vi "Remove Keys.vi"(8 "error in (no error)":errorcluster) -> (0 "error out":errorcluster, 3 "text":string)   [LabVIEW 2017, in "csm-ini-variable-addon.lvclass"]
uses:
  csm-ini-variable-addon.lvclass
  INI-Static-Variable-Support/LabVIEW-Config/LabVIEW-Config.lvclass
panel:
  out "Section Names After":string[](array[string])
  out "Key Names Before":string[](array[string])
  out "Key Names After":string[](array[string])
  out "Section Names Before":string[](array[string])
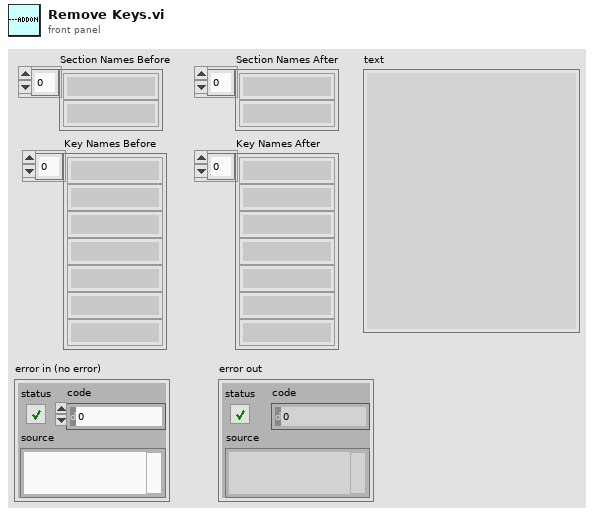
[diagram p1: front panel]
types:
  T1 = typedef "LabVIEW-Config.lvlib/LabVIEW-Config.lvclass/Config.ctl" = cluster{"Path":path, "Lines":string[], "Tokens":T2[], "Modified?":bool, "Cache":cluster{"Valid?":bool, "Key Information":T3[]}}
  T2 = typedef "LabVIEW-Config.lvlib/LabVIEW-Config.lvclass/LineToken.ctl" = enum8{"comment", "section", "key", "more"}
  T3 = typedef "LabVIEW-Config.lvlib/LabVIEW-Config.lvclass/KeyInfo.ctl" = cluster{"Key Indexes":cluster{"Indexes":i32[]}[], "Session Found?":bool, "Key found?":bool, "Session Index":i32}
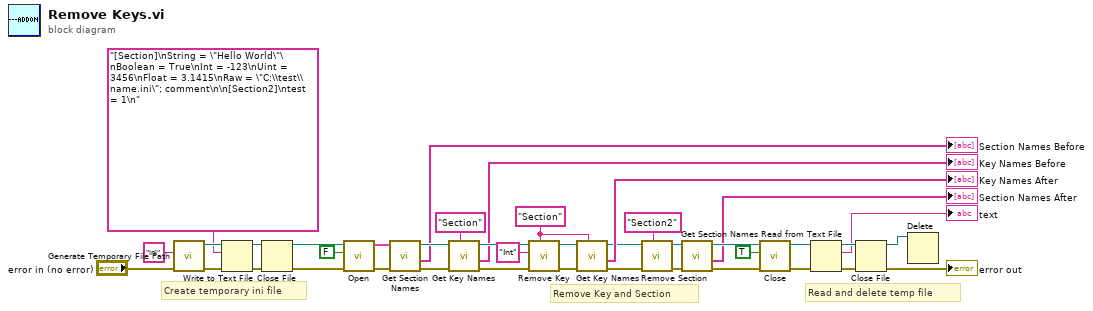
[diagram p0: block diagram]
diagram:
  w1 = "Section"
  # "Remove Key and Section"
  # "Read and delete temp file"
  # "Create temporary ini file"
  n1 = call <vilib>:"Generate Temporary File Path.vi"("error in (no error)"="error in (no error)", "Temporary File Extension (tmp)"="ini") -> ("error out"=w36:errorcluster, "Unique Temporary File Path"=w33:path)  [unwired: 8 in]
  n2 = Write to Text File(file (use dialog)=w33, text="[Section]\nString = \"Hello World\"\nBoolean = True\nInt = -123\nUint = 3456\nFloat = 3.1415\nRaw = \"C:\\test\\name.ini\"; comment\n\n[Section2]\ntest = 1\n", error in=w36) -> (refnum out=w32:refnum<file>, error out=w34:errorcluster)  [unwired: 1 in, 1 out]
  n3 = Close File(refnum=w32, error in=w34) -> (path=w28:path, error out=w29:errorcluster)
  n4 = call "Open.vi"("error in (no error)"=w29, "Create if not exists? (T)"=FALSE, "Path"=w28) -> ("error out"=w38:errorcluster, "Config"=w24:T1)  [unwired: 5 in, 2 out]
  n5 = call "Get Section Names.vi"("error in (no error)"=w38, "Config in"=w24) -> ("error out"=w27:errorcluster, "Section Names"=→"Section Names Before":string[], "Config out"=w20:refnum<class "LabVIEW-Config.lvclass">)  [unwired: 7 in]
  n6 = call "Get Key Names.vi"("Section Name"="Section", "error in (no error)"=w27, "Config in"=w20) -> ("error out"=w21:errorcluster, "Key Names"=→"Key Names Before":string[], "Config out"=w19:refnum<class "LabVIEW-Config.lvclass">)  [unwired: 5 in, 1 out]
  n7 = call "Remove Key.vi"("Section Name"=w1, "error in (no error)"=w21, "Key Name"="Int", "Config in"=w19) -> ("error out"=w23:errorcluster, "Config out"=w22:refnum<class "LabVIEW-Config.lvclass">)  [unwired: 5 in, 1 out]
  n8 = call "Get Key Names.vi"("Section Name"=w1, "error in (no error)"=w23, "Config in"=w22) -> ("error out"=w26:errorcluster, "Key Names"=→"Key Names After":string[], "Config out"=w13:refnum<class "LabVIEW-Config.lvclass">)  [unwired: 5 in, 1 out]
  n9 = call "Remove Section.vi"("Section Name"="Section2", "error in (no error)"=w26, "Config in"=w13) -> ("error out"=w14:errorcluster, "Config out"=w10:refnum<class "LabVIEW-Config.lvclass">)  [unwired: 6 in, 1 out]
  n10 = call "Get Section Names.vi"("error in (no error)"=w14, "Config in"=w10) -> ("error out"=w11:errorcluster, "Section Names"=→"Section Names After":string[], "Config out"=w9:refnum<class "LabVIEW-Config.lvclass">)  [unwired: 7 in]
  n11 = call "Close.vi"("error in (no error)"=w11, "Write if modified? (T)"=TRUE, "Config"=w9) -> ("error out"=w30:errorcluster, "Path"=w6:path)  [unwired: 7 in]
  n12 = Read from Text File(file (use dialog)=w6, error in=w30) -> (refnum out=w4:refnum<file>, text=→"text":string, error out=w7:errorcluster)  [unwired: 2 in, 1 out]
  n13 = Close File(refnum=w4, error in=w7) -> (path=w3:path, error out=→"error out":errorcluster)
  n14 = Delete(path (use dialog)=w3) -> ()  [unwired: 4 in, 3 out]
